vi "ExportVIContent.vi"(6 "CodeSchema":string, 10 "ILabVIEWItem in":refnum<class "ILabVIEWItem.lvclass">, 11 "CGrapherDGML in":refnum<class "CGrapherDGML.lvclass">) -> (1 "Links":T1, 2 "Nodes":T1, 3 "CGrapherDGML":refnum<class "CGrapherDGML.lvclass">)   [LabVIEW 2020, in "DefaultExtensions.lvlib" / "CGrapherDGML.lvclass"]
uses:
  CGrapherDGML.lvclass
  LabVIEWObjectInterfaces/ILabVIEWItem/ILabVIEWItem.lvclass
  LabVIEWItem/CLabVIEWItem/ConnectionSet.ctl
  CGrapherDGML.lvclass/CGrapherDGML.ctl
  LabVIEWItem/CLabVIEWItem/CLabVIEWItem.lvclass
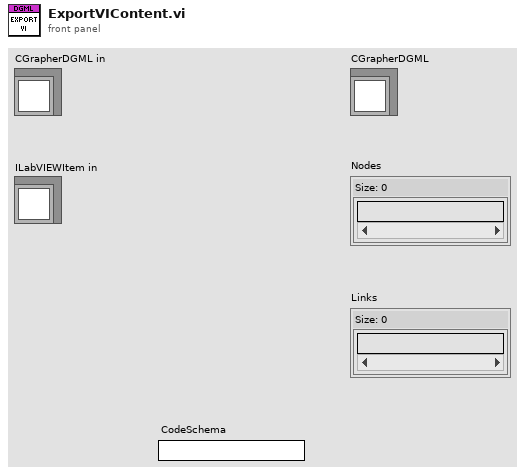
[diagram p1: front panel]
types:
  T1 = typedef "LabVIEWItem.lvlib/CLabVIEWItem.lvclass/ConnectionSet.ctl" = set{string}
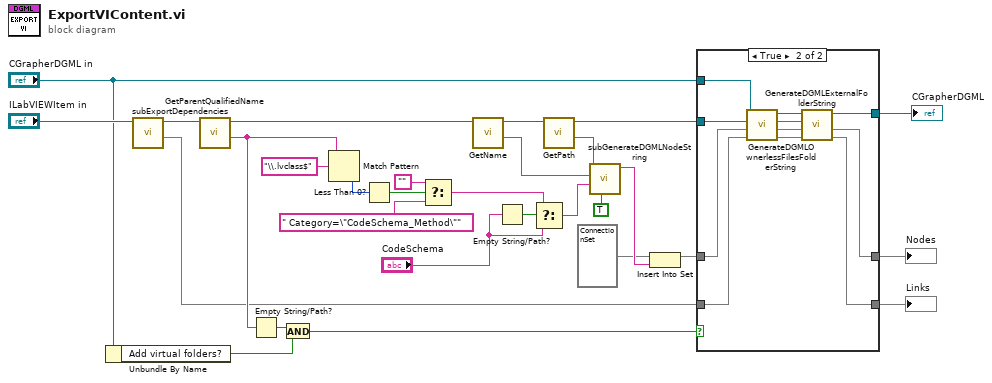
[diagram p0: block diagram]
diagram:
  n1 = Unbundle By Name("CGrapherDGML in") -> ("Add virtual folders?"=w3:bool)
  n2 = call "subExportDependencies.vi"("ILabVIEWItem in"="ILabVIEWItem in") -> ("Links"=w16:T1, "ILabVIEWItem out"=w28:refnum<class "ILabVIEWItem.lvclass">)  [unwired: 8 in, 1 out]
  n3 = call-dynamic "GetParentQualifiedName.vi"("ILabVIEWItem in"=w28) -> ("Name"=w19:string, "ILabVIEWItem out"=w27:refnum<class "ILabVIEWItem.lvclass">)  [unwired: 8 in, 1 out]
  n4 = Empty String/Path?(string/path=w19) -> (empty?=w14:bool)
  n5 = And(x=w14, y=w3) -> (x .and. y?=w13:bool)
  n6 = Match Pattern(string=w19, regular expression="\\.lvclass$") -> (offset past match=w25:i32)  [unwired: 1 in, 3 out]
  n7 = Less Than 0?(x=w25) -> (x < 0?=w24:bool)
  n8 = Select(t="", s=w24, f=" Category=\"CodeSchema_Method\"") -> (s? t:f=w21:string)
  n9 = call-dynamic "GetName.vi"("ILabVIEWItem in"=w27) -> ("Name"=w12:string, "ILabVIEWItem out"=w5:refnum<class "ILabVIEWItem.lvclass">)  [unwired: 8 in, 1 out]
  n10 = Empty String/Path?(string/path="CodeSchema") -> (empty?=w20:bool)
  n11 = Select(t=w21, s=w20, f="CodeSchema") -> (s? t:f=w11:string)
  n12 = call-dynamic "GetPath.vi"("ILabVIEWItem in"=w5) -> ("Path"=w9:string, "ILabVIEWItem out"=w8:refnum<class "ILabVIEWItem.lvclass">)  [unwired: 8 in, 1 out]
  n13 = call "subGenerateDGMLNodeString.vi"("Container empty?"=TRUE, "Code schema"=w11, "Label"=w12, "Id"=w9) -> ("Node string"=w10:string)  [unwired: 7 in]
  n14 = Insert Into Set(10:w10, 11:T1 {} ("Links")) -> (3:w18:T1)  [unwired: 1 out]
  n15 = case shown="True" w13 {
    tunnel: w16 -> [w31 w42]
    tunnel: [w31 w33] -> w15
    tunnel: w18 -> [w32 w41]
    tunnel: [w32 w34] -> w17
    tunnel: w8 -> [_ w40]
    tunnel: "CGrapherDGML in" -> [w30 w36]
    tunnel: [w30 w35] -> w1
    frame False {
    }
    frame True {
      n16 = call-dynamic "GenerateDGMLOwnerlessFilesFolderString.vi"("Links in"=w42, "Nodes in"=w41, "ILabVIEWItem in"=w40, "CGrapherDGML in"=w36) -> ("Links"=w38:T1, "Nodes"=w39:T1, "Path"=w43:string, "CGrapherDGML"=w37:refnum<class "CGrapherDGML.lvclass">)  [unwired: 4 in]
      n17 = call-dynamic "GenerateDGMLExternalFolderString.vi"("Links in"=w38, "Nodes in"=w39, "Path in"=w43, "CGrapherDGML in"=w37) -> ("Links"=w33:T1, "Nodes"=w34:T1, "CGrapherDGML"=w35:refnum<class "CGrapherDGML.lvclass">)  [unwired: 5 in]
    }
  }
  "Nodes" <- w17
  "Links" <- w15
  "CGrapherDGML" <- w1
